vi "File Save Header to FA File.vi"(6 "BPM and PS selection":T1, 7 "Acquisition period (us)":u32, 8 "error in (no error)":errorcluster, 9 "PS Reading Names":string[](array[string]), 10 "BPM Reading Names":string[](array[string]), 11 "FA File Reference":refnum<file>) -> (0 "error out":errorcluster, 3 "FA File Reference out":refnum<file>)   [LabVIEW 2011, in "File VIs.lvlib"]
uses:
  File VIs.lvlib
  Types Definitions/Type BPM and PS select cluster.ctl
  Type Definitions.lvlib
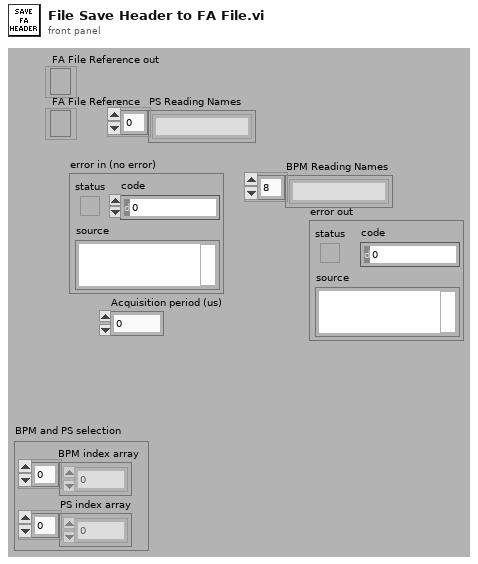
[diagram p1: front panel]
types:
  T1 = typedef "Type Definitions.lvlib/Type BPM and PS select cluster.ctl" = cluster{"BPM index array":u32[], "PS index array ":u32[]}
  T2 = enum16{"big-endian, network order", "native, host order", "little-endian"}
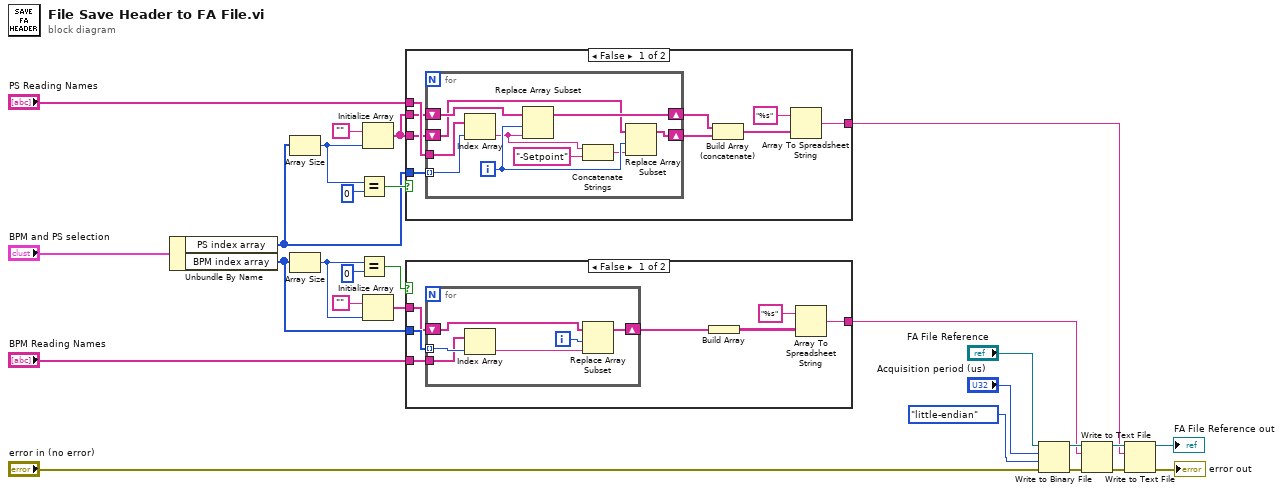
[diagram p0: block diagram]
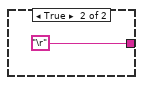
[diagram p2: hidden frame]
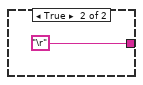
[diagram p3: hidden frame]
diagram:
  n1 = Unbundle By Name("BPM and PS selection") -> ("PS index array"=w8:u32[], "BPM index array"=w17:u32[])
  n2 = Array Size(array=w8) -> (size(s)=w3:i32)
  n3 = Array Size(array=w17) -> (size(s)=w4:i32)
  n4 = Equal?(x=w3, y=0) -> (x = y?=w9:bool)
  n5 = Equal?(x=w4, y=0) -> (x = y?=w14:bool)
  n6 = Initialize Array("", w3) -> (w10:string[])
  n7 = Initialize Array("", w4) -> (w18:string[])
  n8 = case shown="False" w9 {
    tunnel: "PS Reading Names" -> [w36 _]
    tunnel: w8 -> [w35 _]
    tunnel: w10 -> [w34 _]
    tunnel: w10 -> [w33 _]
    tunnel: [w28 "\r"] -> w6
    frame False {
      n9 = for {
        tunnel: w36 -> [w43]
        tunnel: w35 -> [w44] mode=indexing
        shift-right: [w45] -> w30
        shift-left: w34 -> [w46]
        shift-right: [w42] -> w29
        shift-left: w33 -> [w40]
        i -> [w41]
        n10 = Index Array(array=w43, index=w44) -> (element=w37:string)
        n11 = Replace Array Subset(array=w46, new element=w37, index=w41) -> (w45:string[])
        n12 = Concatenate Strings(w37, "-Setpoint") -> (w39:string)
        n13 = Replace Array Subset(array=w40, new element=w39, index=w41) -> (w42:string[])
      }
      n14 = Build Array (concatenate)(w30, w29) -> (w32:string[])
      n15 = Array To Spreadsheet String(array=w32, 3:"%s" ("format string")) -> (spreadsheet string=w28:string)  [unwired: 1 in]
    }
    frame True {
    }
  }
  n16 = case shown="False" w14 {
    tunnel: "BPM Reading Names" -> [w54 _]
    tunnel: w17 -> [w53 _]
    tunnel: w18 -> [w52 _]
    tunnel: [w48 "\r"] -> w5
    frame False {
      n17 = for {
        tunnel: w54 -> [w56]
        tunnel: w53 -> [w57] mode=indexing
        shift-right: [w58] -> w50
        shift-left: w52 -> [w60]
        i -> [w59]
        n18 = Index Array(array=w56, index=w57) -> (element=w55:string)
        n19 = Replace Array Subset(array=w60, new element=w55, index=w59) -> (w58:string[])
      }
      n20 = Build Array(w50) -> (w49:string[][])
      n21 = Array To Spreadsheet String(array=w49, 3:"%s" ("format string")) -> (spreadsheet string=w48:string)  [unwired: 1 in]
    }
    frame True {
    }
  }
  n22 = Write to Binary File(file (use dialog)="FA File Reference", data="Acquisition period (us)", error in="error in (no error)", 9:T2."little-endian" ("byte order (0:big-endian, network order)")) -> (refnum out=w23:refnum<file>, error out=w21:errorcluster)  [unwired: 2 in, 1 out]
  n23 = Write to Text File(file (use dialog)=w23, text=w5, error in=w21) -> (refnum out=w26:refnum<file>, error out=w27:errorcluster)  [unwired: 1 in, 1 out]
  n24 = Write to Text File(file (use dialog)=w26, text=w6, error in=w27) -> (refnum out=→"FA File Reference out":refnum<file>, error out=→"error out":errorcluster)  [unwired: 1 in, 1 out]
